vi "Open Gates.vi"(8 "error in (no error)":errorcluster, 11 "gate":T1) -> (0 "error out":errorcluster, 3 "gate out":T1)   [LabVIEW 2015, in "Gates.lvlib"]
doc: "Opens referenced gate."
uses:
  Gates.lvlib
  Gate.ctl
  Gate Pass.ctl
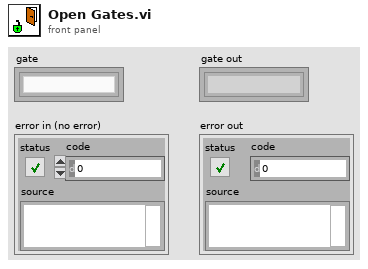
[diagram p1: front panel]
types:
  T1 = typedef "Gates.lvlib/Gate.ctl" = refnum<k1>
  T2 = typedef "Gates.lvlib/Gate Pass.ctl" = refnum<k1>
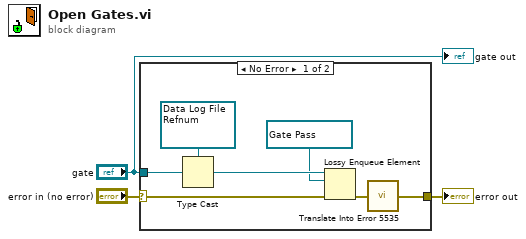
[diagram p0: block diagram]
diagram:
  n1 = case shown="No Error" "error in (no error)" {
    selector: "error in (no error)" -> [w8 w11]
    tunnel: "gate" -> [w9 _]
    tunnel: [w4 w11] -> w1
    frame No Error {
      w6 = T2 refnum items=["Gate Pass"] ("Data Log File Refnum")
      w10 = refnum<queue> refnum items=["Gate Pass"] ("queue out")
      n2 = Type Cast(type=w10, x=w9) -> (*(type *) &x=w7:refnum<queue>)
      n3 = Lossy Enqueue Element(queue=w7, element=w6, error in (no error)=w8) -> (error out=w5:errorcluster)  [unwired: 3 out]
      n4 = call "Translate Into Error 5535.vi"("error in (no error)"=w5) -> ("error out"=w4:errorcluster)  [unwired: 1 in]
    }
    frame Error {
    }
  }
  "error out" <- w1
  "gate out" <- "gate"
